vi "Recursive Build Path.vi"(2 "file name":string, 3 "Path":path) -> (0 "file path name":path)   [LabVIEW 2017]
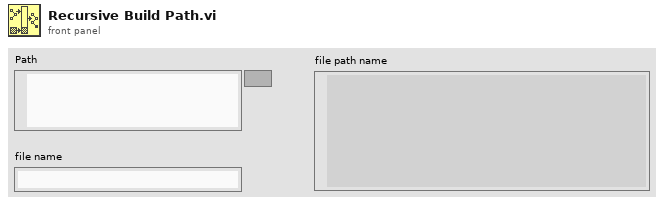
[diagram p1: front panel]
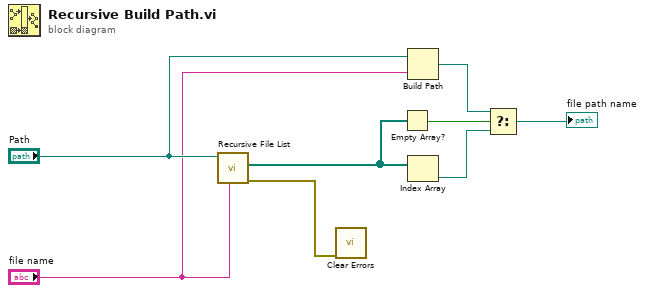
[diagram p0: block diagram]
diagram:
  n1 = call <vilib>:"Recursive File List.vi"("pattern"="file name", "Folder Path"="Path") -> ("error out"=w1:errorcluster, "All Files in Dir"=w8:path[])  [unwired: 5 in, 3 out]
  n2 = call <vilib>:"Clear Errors.vi"("error in (no error)"=w1) -> ()  [unwired: 5 in, 2 out]
  n3 = Empty Array?(array=w8) -> (empty?=w7:bool)
  n4 = Build Path(base path="Path", name or relative path="file name") -> (appended path=w5:path)
  n5 = Index Array(array=w8) -> (element=w6:path)  [unwired: 1 in]
  n6 = Select(t=w5, s=w7, f=w6) -> (s? t:f=→"file path name":path)
